vi "GalvoCheck.vi"(0 "Reset galvo position ?":bool, 1 "scan frequency":dbl[unit]=1.0 min=1.0, 2 "amplitude in":dbl[unit]=1.0 format="%0.2f", 3 "cycles":u32=1 min=1) -> (9 "stimulus and response":waveform(dbl)[](graph))   [LabVIEW 2010]
uses:
  <vilib>/DAQmx/write.llb/DAQmx Write (Analog 1D DBL 1Chan NSamp).vi
  <vilib>/DAQmx/read.llb/DAQmx Read (Analog 1D DBL 1Chan NSamp).vi
  <vilib>/DAQmx/create/channels.llb/DAQmx Create Channel (AI-Voltage-Basic).vi
  <vilib>/DAQmx/configure/timing.llb/DAQmx Timing (Sample Clock).vi
  <vilib>/DAQmx/configure/trigger.llb/DAQmx Start Trigger (Digital Edge).vi
  <vilib>/DAQmx/create/channels.llb/DAQmx Create Channel (AO-Voltage-Basic).vi
  <vilib>/addons/System Identification/Data Preprocess.llb/SI Split Signal (SISO Waveform).vi
  <vilib>/measure/mascope.llb/Amplitude and Levels 1 chan.vi
  <vilib>/daqmx/miscellaneous.llb/DAQmx Fill In Error Info.vi
  <vilib>/addons/System Identification/NI_SysID.lvlib
  <vilib>/addons/System Identification/Data Preprocess.llb/SI Normalize (SISO Waveform).vi
  <vilib>/addons/System Identification/Model Analysis.llb/SI Model Simulation (SISO Waveform).vi
  <vilib>/addons/System Identification/Parametric Estimation.llb/SI Estimate State-Space Model (SISO Waveform).vi
  <vilib>/Analysis/NI_AALPro.lvlib
  <vilib>/measure/NI_MAPro.lvlib
panel:
  in  "position plot scale factor":dbl
  out "center position (V)":dbl
  out "position/command scaling factor":dbl[unit]
  out "min position (V)":dbl format="%.2g"
  out "max position (V)":dbl format="%.2g"
  out "position amplitude (V)":dbl format="%.2p"
  in  "number of states":i32=10
  out "State-space model evaluation":waveform(dbl)[](graph)
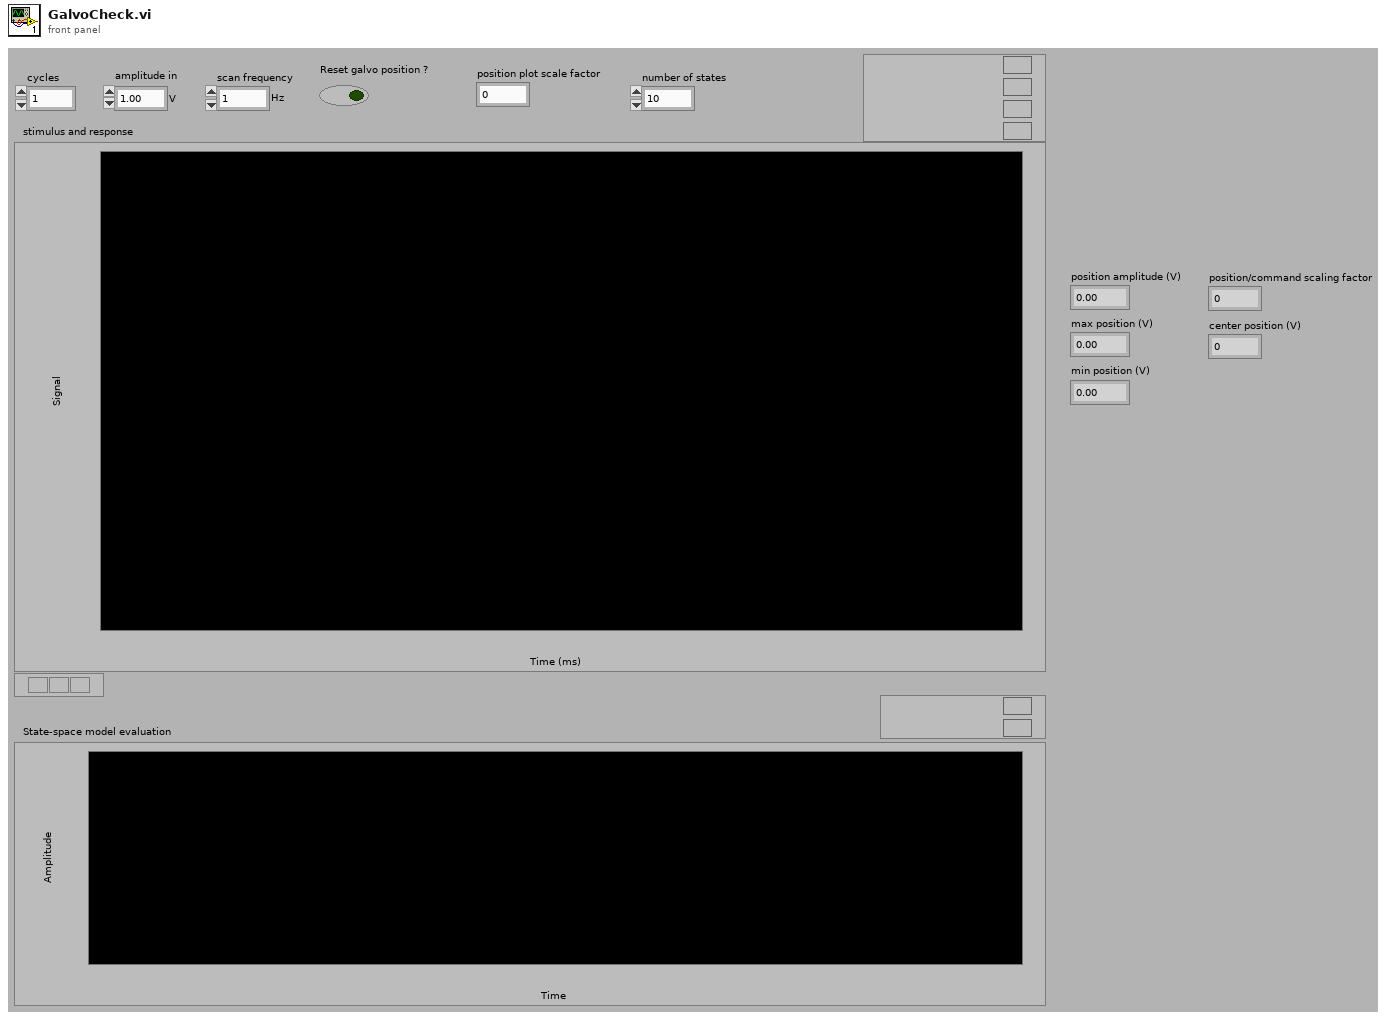
[diagram p1: front panel]
types:
  T1 = typedef "NI_SysID.lvlib/si_generic model.ctl" = cluster{"attributes":cluster{"version":string, "model type":T2, "input names":string[], "output names":string[], "notes":string}, "coefficients":cluster{"A ":dbl[][][], "B":dbl[][][], "F":dbl[][][], "C":dbl[][][], "D":dbl[][][]}, "std deviations":cluster{"A ":dbl[][][], "B":dbl[][][], "F":dbl[][][], "C":dbl[][][], "D":dbl[][][]}, "coefficients covariance":dbl[][][], "noise variance":dbl[][], "fs":dbl, "system info":cluster{"number of inputs":i32, "number of outputs":i32, "A order":i32[][], "B order":i32[][], "F order":i32[][], "C order":i32[][], "D order":i32[][], "Delays":i32[][]}, "kalman gain":dbl[][], "initial state":dbl[], "trans func":cluster{"betas":dbl[], "alphas":dbl[]}[][], "zeros-poles":cluster{"zeros":cdb[], "poles":cdb[], "gain":dbl}[][], "std of trans func":cluster{"betas":dbl[], "alphas":dbl[]}[][], "std of zeros-poles":cluster{"zeros":cdb[], "poles":cdb[], "gain":dbl}[][], "trans func (noise)":cluster{"betas":dbl[], "alphas":dbl[]}[][], "std of trans func (noise)":cluster{"betas":dbl[], "alphas":dbl[]}[][], "zeros-poles (noise)":cluster{"zeros":cdb[], "poles":cdb[], "gain":dbl}[][], "std of zeros-poles (noise)":cluster{"zeros":cdb[], "poles":cdb[], "gain":dbl}[][], "Symbolic State Space Model":cluster{"Symbolic A":string[][], "Symbolic B":string[][], "Symbolic C":string[][], "Symbolic D":string[][], "Symbolic K":string[][], "Symbolic Initial State":string[]}, "delay":dbl[][], "variables":T3, "grey trans func spec":cluster{"orders of TF model":cluster{" num order":i32, "den order":i32}, "# of zeros/poles at origin":cluster{"zeros/poles":u16, "number ":i32}, "delay initial?":bool, "gain initial?":bool}}
  T2 = typedef "NI_SysID.lvlib/SI Model Type.ctl" = u16
  T3 = typedef "NI_SysID.lvlib/si_variables.ctl" = cluster{"name":string, "initial guess":dbl, "upper limit":dbl, "lower limit":dbl, "value":dbl}[]
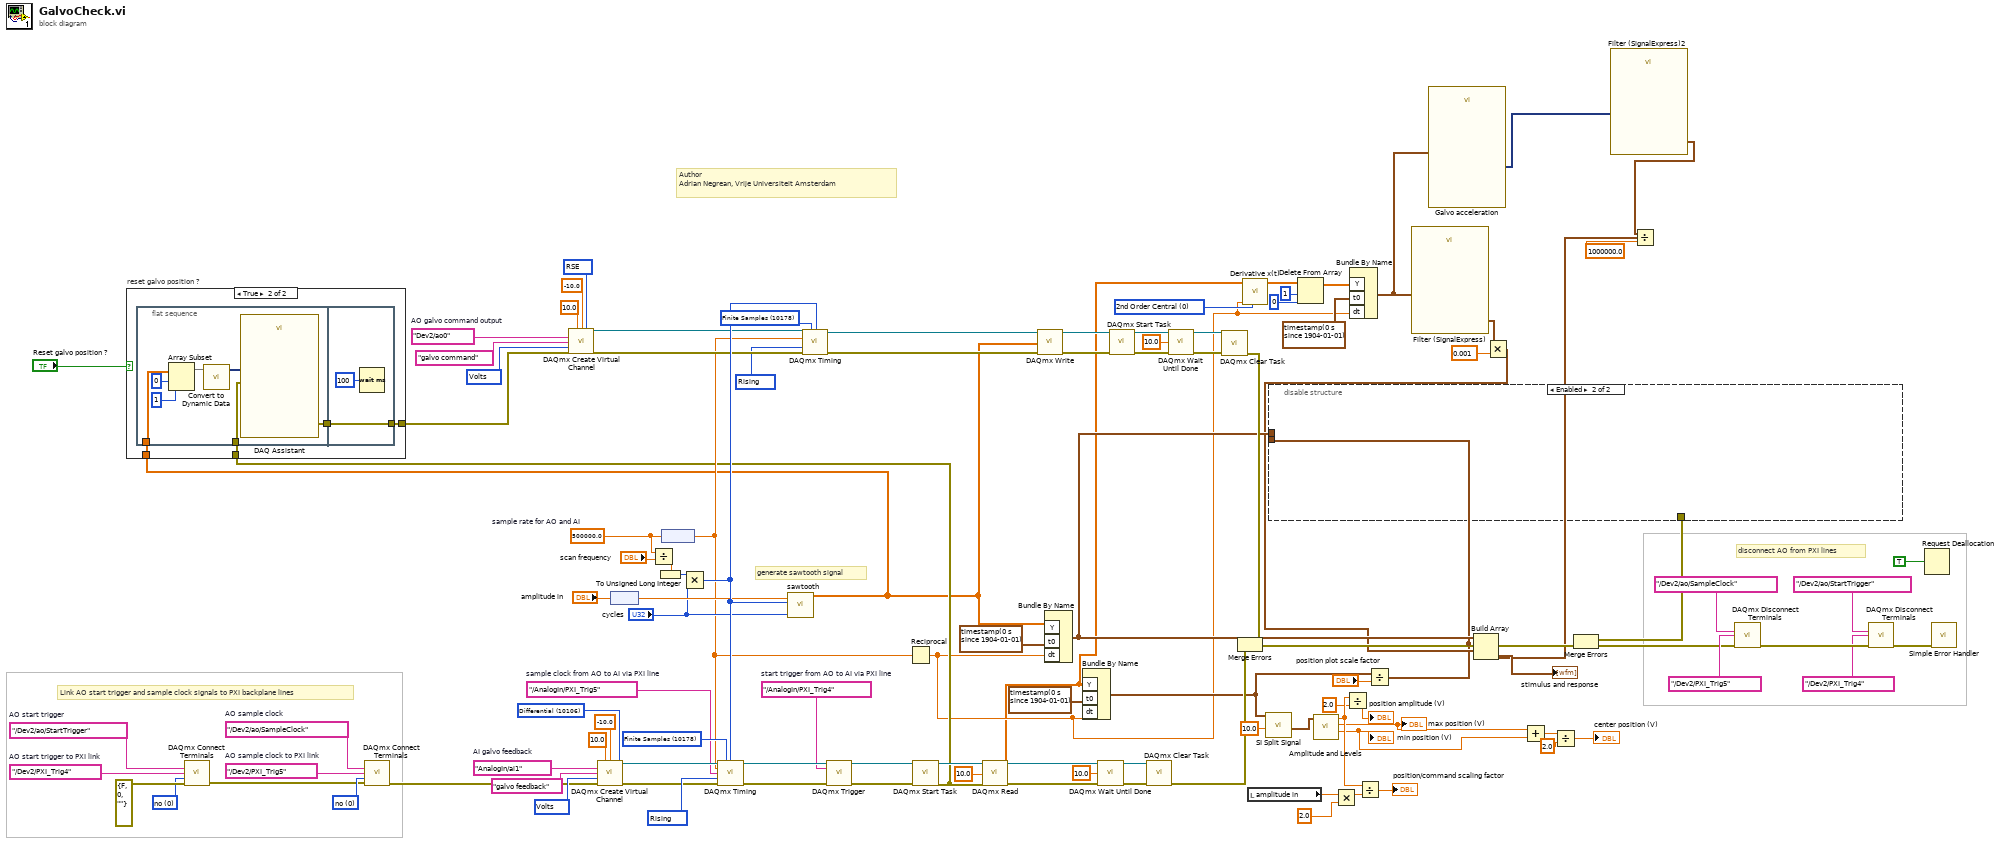
[diagram p0: block diagram]
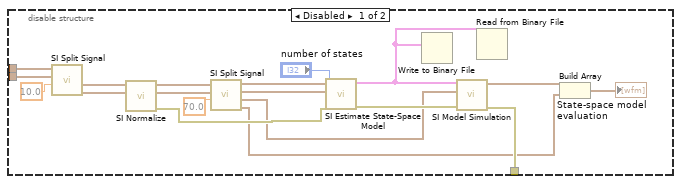
[diagram p2: hidden frame]
diagram:
  w29 = u16 0 items=["2nd Order Central", "4th Order Central", "Forward", "Backward"] ("method")
  w66 = tag "Dev2/ao0"  # AO galvo command output
  w79 = dbl[unit] 500000.0  # sample rate for AO and AI
  w105 = tag "AnalogIn/ai1"  # AI galvo feedback
  w53 = tag "/AnalogIn/PXI_Trig4"  # start trigger from AO to AI via PXI line
  w97 = tag "/AnalogIn/PXI_Trig5"  # sample clock from AO to AI via PXI line
  w57 = 10178 items=["Finite Samples"=10178, "Continuous Samples"=10123, "Hardware Timed Single Point"=12522] ("command generation type")
  w58 = 10280 items=["Rising"=10280, "Falling"=10171] ("active edge")
  w63 = 10083 items=["Default"=-1, "RSE"=10083, "Differential"=10106, "Pseudodifferential"=12529] ("output terminal configuration")
  w64 = 10348 items=["Volts"=10348, "From Custom Scale"=10065] ("units")
  w96 = 10280 items=["Rising"=10280, "Falling"=10171] ("active edge")
  w98 = 10178 items=["Finite Samples"=10178, "Continuous Samples"=10123, "Hardware Timed Single Point"=12522] ("sample mode")
  w100 = 10106 items=["default"=-1, "RSE"=10083, "NRSE"=10078, "Differential"=10106, "Pseudodifferential"=12529] ("input terminal configuration")
  w103 = 10348 items=["Volts"=10348, "From Custom Scale"=10065] ("units")
  w48 = tag "/Dev2/ao/StartTrigger"  # AO start trigger
  w108 = 0 items=["no", "yes"] ("invert polarity")
  w110 = tag "/Dev2/PXI_Trig4"  # AO start trigger to PXI link
  w111 = tag "/Dev2/ao/SampleClock"  # AO sample clock
  w112 = 0 items=["no", "yes"] ("invert polarity")
  w113 = tag "/Dev2/PXI_Trig5"  # AO sample clock to PXI link
  # "generate sawtooth signal"
  # "disconnect AO from PXI lines"
  # "Link AO start trigger and sample clock signals to PXI backplane lines"
  # "Author\nAdrian Negrean, Vrije Universiteit Amsterdam"
  n1 = call <vilib>:"DAQmx Connect Terminals.vi"("source terminal"=w48, "destination terminal"=w110, "invert polarity"=w108, "error in"=errorcluster {"status"=FALSE, "code"=0, "source"=""}) -> ("error out"=w107:errorcluster)  [unwired: 11 in]
  n2 = call <vilib>:"DAQmx Connect Terminals.vi"("source terminal"=w111, "destination terminal"=w113, "invert polarity"=w112, "error in"=w107) -> ("error out"=w84:errorcluster)  [unwired: 11 in]
  n3 = call-poly <vilib>:"DAQmx Create Virtual Channel.vi"("maximum value"=10.0, "minimum value"=-10.0, "input terminal configuration"=w100, "physical channels"=w105, "name to assign"="galvo feedback", "units"=w103, "error in"=w84) -> ("task out"=w99:refnum<k21>, "error out"=w82:errorcluster)  [unwired: 7 in]
  n4 = node("amplitude in") -> (w80:dbl)
  n5 = Divide(x=w79, y="scan frequency") -> (x/y=w76:dbl)
  n6 = To Unsigned Long Integer(number=w76) -> (unsigned 32bit integer=w75:u32)
  n7 = node(w79) -> (w46:dbl)
  n8 = Multiply(x=w75, y="cycles") -> (x*y=w106:u32)
  n9 = call-poly <vilib>:"DAQmx Timing.vi"("task/channels in"=w99, "sample mode"=w98, "samples per channel"=w106, "rate"=w46, "source"=w97, "active edge"=w96, "error in"=w82) -> ("task out"=w93:refnum<k21>, "error out"=w92:errorcluster)  [unwired: 7 in]
  n10 = call "sawtooth.vi"("cycles"="cycles", "samples"=w106, "amplitude in"=w80) -> ("sawtooth signal"=w35:dbl[])  [unwired: 8 in]
  n11 = call-poly <vilib>:"DAQmx Trigger.vi"("task/channels in"=w93, "source"=w53, "error in"=w92) -> ("task out"=w91:refnum<k21>, "error out"=w83:errorcluster)  [unwired: 11 in]
  n12 = Reciprocal(x=w46) -> (1/x=w7:dbl)
  n13 = call <vilib>:"DAQmx Start Task.vi"("task/channels in"=w91, "error in"=w83) -> ("task out"=w94:refnum<k21>, "error out"=w41:errorcluster)  [unwired: 12 in]
  n14 = case "reset galvo position ?" shown="True" "Reset galvo position ?" {
    tunnel: w41 -> [w114 w118]
    tunnel: [w114 w117] -> w40
    tunnel: w35 -> [_ w116]
    frame False {
    }
    frame True {
      n15 = flat-sequence {
        tunnel: w118 -> [w121]
        tunnel: w116 -> [w119]
        tunnel: [w120] -> w115
        tunnel: [w127] -> w117
        tunnel: w115 -> [w127]
        frame #0 {
          n16 = Array Subset(array=w119, index=0, length=1) -> (w123:dbl[])
          n17 = call "Convert to Dynamic Data"("Array"=w123) -> ("Dynamic Data Type"=w122:dynamicdata)  [unwired: 3 in]
          n18 = call "DAQ Assistant"("data"=w122, "error in"=w121) -> ("error out"=w120:errorcluster)  [unwired: 16 in, 1 out]
        }
        frame #1 {
          n19 = Wait (ms)(milliseconds to wait=u32 100) -> ()  [unwired: 1 out]
        }
      }
    }
  }
  n20 = call-poly <vilib>:"DAQmx Create Virtual Channel.vi"("maximum value"=10.0, "minimum value"=-10.0, "output terminal configuration"=w63, "physical channels"=w66, "name to assign"="galvo command", "units"=w64, "error in"=w40) -> ("task out"=w60:refnum<k21>, "error out"=w59:errorcluster)  [unwired: 7 in]
  n21 = call-poly <vilib>:"DAQmx Timing.vi"("task/channels in"=w60, "sample mode"=w57, "samples per channel"=w106, "rate"=w46, "active edge"=w58, "error in"=w59) -> ("task out"=w56:refnum<k21>, "error out"=w55:errorcluster)  [unwired: 8 in]
  n22 = call-poly <vilib>:"DAQmx Read.vi"("task/channels in"=w94, "timeout"=10.0, "error in"=w41) -> ("task out"=w90:refnum<k21>, "data"=w6:dbl[], "error out"=w74:errorcluster)  [unwired: 10 in]
  n23 = call-poly <vilib>:"DAQmx Write.vi"("task/channels in"=w56, "data"=w35, "error in"=w55) -> ("task out"=w73:refnum<k21>, "error out"=w72:errorcluster)  [unwired: 10 in, 1 out]
  n24 = Bundle By Name("Y"=w35, "t0"=timestamp(0 s since 1904-01-01), "dt"=w7) -> (w34:waveform(dbl))  [unwired: 1 in]
  n25 = Bundle By Name("Y"=w6, "t0"=timestamp(0 s since 1904-01-01), "dt"=w7) -> (w13:waveform(dbl))  [unwired: 1 in]
  n26 = call <vilib>:"DAQmx Wait Until Done.vi"("task/channels in"=w90, "timeout (sec)"=10.0, "error in"=w74) -> ("task out"=w89:refnum<k21>, "error out"=w88:errorcluster)  [unwired: 11 in]
  n27 = call <vilib>:"DAQmx Start Task.vi"("task/channels in"=w73, "error in"=w72) -> ("task out"=w71:refnum<k21>, "error out"=w69:errorcluster)  [unwired: 12 in]
  n28 = call <vilib>:"DAQmx Clear Task.vi"("task in"=w89, "error in"=w88) -> ("error out"=w54:errorcluster)  [unwired: 13 in]
  n29 = call <vilib>:"DAQmx Wait Until Done.vi"("task/channels in"=w71, "timeout (sec)"=10.0, "error in"=w69) -> ("task out"=w70:refnum<k21>, "error out"=w68:errorcluster)  [unwired: 11 in]
  n30 = call <vilib>:"DAQmx Clear Task.vi"("task in"=w70, "error in"=w68) -> ("error out"=w42:errorcluster)  [unwired: 13 in]
  n31 = Merge Errors(w42, w54) -> (w38:errorcluster)
  n32 = call <vilib>:"Derivative x(t).vi"("method"=w29, "dt"=w7, "X"=w6) -> ("dX/dt"=w8:dbl[])  [unwired: 7 in, 1 out]
  n33 = local read "amplitude in"() -> (w25:dbl[unit])
  n34 = call-poly <vilib>:"SI Split Signal.vi"("1st portion (%)"=10.0, "stimulus signal in"=w13) -> ("stimulus signal 2"=w14:waveform(dbl))  [unwired: 6 in, 3 out]
  n35 = Delete From Array(array=w8, length=1, index=0) -> (array with subset deleted=w30:dbl[])  [unwired: 1 out]
  n36 = call-poly <vilib>:"Amplitude and Levels.vi"("signal in"=w14) -> ("low state level"=w19:dbl, "high state level"=w20:dbl, "amplitude"=w24:dbl)  [unwired: 7 in, 1 out]
  "max position (V)" <- w20
  "min position (V)" <- w19
  n37 = Multiply(x=w25, y=dbl[unit] 2.0) -> (x*y=w23:dbl[unit])
  n38 = Divide(x=w24, y=2.0) -> (x/y=→"position amplitude (V)":dbl)
  n39 = Bundle By Name("Y"=w30, "t0"=timestamp(0 s since 1904-01-01), "dt"=w7) -> (w5:waveform(dbl))  [unwired: 1 in]
  n40 = Divide(x=w24, y=w23) -> (x/y=→"position/command scaling factor":dbl[unit])
  n41 = Divide(x=w13, y="position plot scale factor") -> (x/y=w10:waveform(dbl))
  n42 = disable-structure shown="Enabled" {
    disable-tunnel: [w138 _] -> w39
    disable-tunnel: w34 -> [w130 _]
    disable-tunnel: w10 -> [w129 _]
    frame Disabled {
      n43 = call-poly <vilib>:"SI Split Signal.vi"("1st portion (%)"=10.0, "response signal in"=w129, "stimulus signal in"=w130) -> ("response signal 2"=w132:waveform(dbl), "stimulus signal 2"=w133:waveform(dbl))  [unwired: 5 in, 2 out]
      n44 = call-poly <vilib>:"SI Normalize.vi"("response signal in"=w132, "stimulus signal in"=w133) -> ("error out"=w139:errorcluster, "response signal out"=w144:waveform(dbl), "stimulus signal out"=w145:waveform(dbl))  [unwired: 5 in, 2 out]
      n45 = call-poly <vilib>:"SI Split Signal.vi"("1st portion (%)"=70.0, "response signal in"=w144, "stimulus signal in"=w145) -> ("response signal 2"=w136:waveform(dbl), "stimulus signal 2"=w137:waveform(dbl), "response signal 1"=w134:waveform(dbl), "stimulus signal 1"=w135:waveform(dbl))  [unwired: 5 in]
      n46 = call-poly <vilib>:"SI Estimate State-Space Model.vi"("error in (no error)"=w139, "number of states"="number of states", "response signal"=w134, "stimulus signal"=w135) -> ("error out"=w140:errorcluster, "system model out"=w128:T1)  [unwired: 2 in, 4 out]
      n47 = Write to Binary File(data=w128) -> ()  [unwired: 5 in, 3 out]
      n48 = call-poly <vilib>:"SI Model Simulation.vi"("error in (no error)"=w140, "stimulus signal"=w137, "system model"=w128) -> ("error out"=w138:errorcluster, "response"=w142:waveform(dbl))  [unwired: 6 in, 1 out]
      n49 = Read from Binary File(5:w128) -> ()  [unwired: 5 in, 4 out]
      n50 = Build Array(w142, w136) -> (→"State-space model evaluation":waveform(dbl)[])
    }
    frame Enabled {
    }
  }
  n51 = call "Filter (SignalExpress)"("input signal"=w5) -> ("filtered data"=w27:waveform(dbl))  [unwired: 17 in, 1 out]
  n52 = call "Galvo acceleration"("Signals"=w5) -> ("Result"=w3:dynamicdata)  [unwired: 5 in, 1 out]
  n53 = Multiply(x=w27, y=0.001) -> (x*y=w26:waveform(dbl))
  n54 = Add(x=w20, y=w19) -> (x+y=w17:dbl)
  n55 = Divide(x=w17, y=2.0) -> (x/y=→"center position (V)":dbl)
  n56 = Merge Errors(w39, w38) -> (w37:errorcluster)
  n57 = call "Filter (SignalExpress)2"("input signal"=w3) -> ("filtered data"=w2:waveform(dbl))  [unwired: 17 in, 1 out]
  n58 = Divide(x=w2, y=1000000.0) -> (x/y=w1:waveform(dbl))
  n59 = Build Array(w34, w10, w26, w1) -> (→"stimulus and response":waveform(dbl)[])
  n60 = call <vilib>:"DAQmx Disconnect Terminals.vi"("source terminal"=tag "/Dev2/ao/SampleClock", "destination terminal"=tag "/Dev2/PXI_Trig5", "error in"=w37) -> ("error out"=w86:errorcluster)  [unwired: 12 in]
  n61 = call <vilib>:"DAQmx Disconnect Terminals.vi"("source terminal"=tag "/Dev2/ao/StartTrigger", "destination terminal"=tag "/Dev2/PXI_Trig4", "error in"=w86) -> ("error out"=w85:errorcluster)  [unwired: 12 in]
  n62 = Request Deallocation(TRUE ("flag")) -> ()
  n63 = call <vilib>:"Simple Error Handler.vi"("error in (no error)"=w85) -> ()  [unwired: 4 in, 5 out]
